vi "update gimbal.vi"(8 "error in \n(no error)":errorcluster, 10 "Current Position":T1, 11 "Data":T2) -> (0 "error out":errorcluster, 3 "Data":T2)   [LabVIEW 2015]
doc: "Artificial Horizon.VI\n\nRecieves Pitch Roll and Head, and using a 3D picture control Builds up an artifical horizon similar to that found in aircraft for example."
uses:
  typedefs/gimbal data.ctl
  <vilib>/Utility/miscctls.llb/LV3DPointTypeDef.ctl
  <vilib>/picture/3D Picture Control/NI_3D Picture Control.lvlib
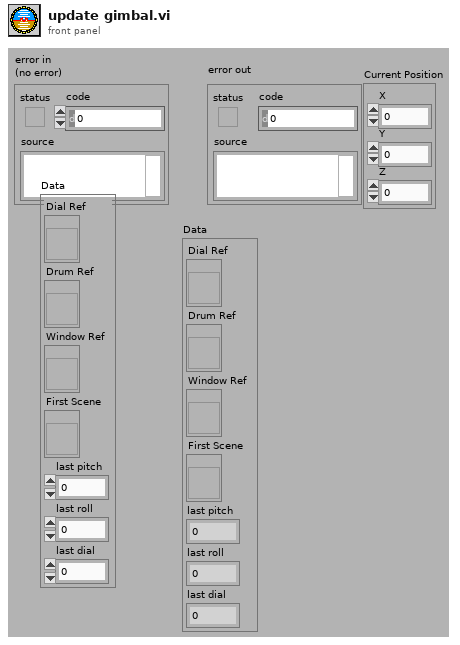
[diagram p1: front panel]
types:
  T1 = typedef "LV3DPointTypeDef.ctl" = cluster{"X":sgl, "Y":sgl, "Z":sgl}
  T2 = typedef "gimbal data.ctl" = cluster{"Dial Ref":refnum<vi>, "Drum Ref":refnum<vi>, "Window Ref":refnum<vi>, "First Scene":refnum<vi>, "last pitch":dbl, "last roll":dbl, "last dial":dbl}
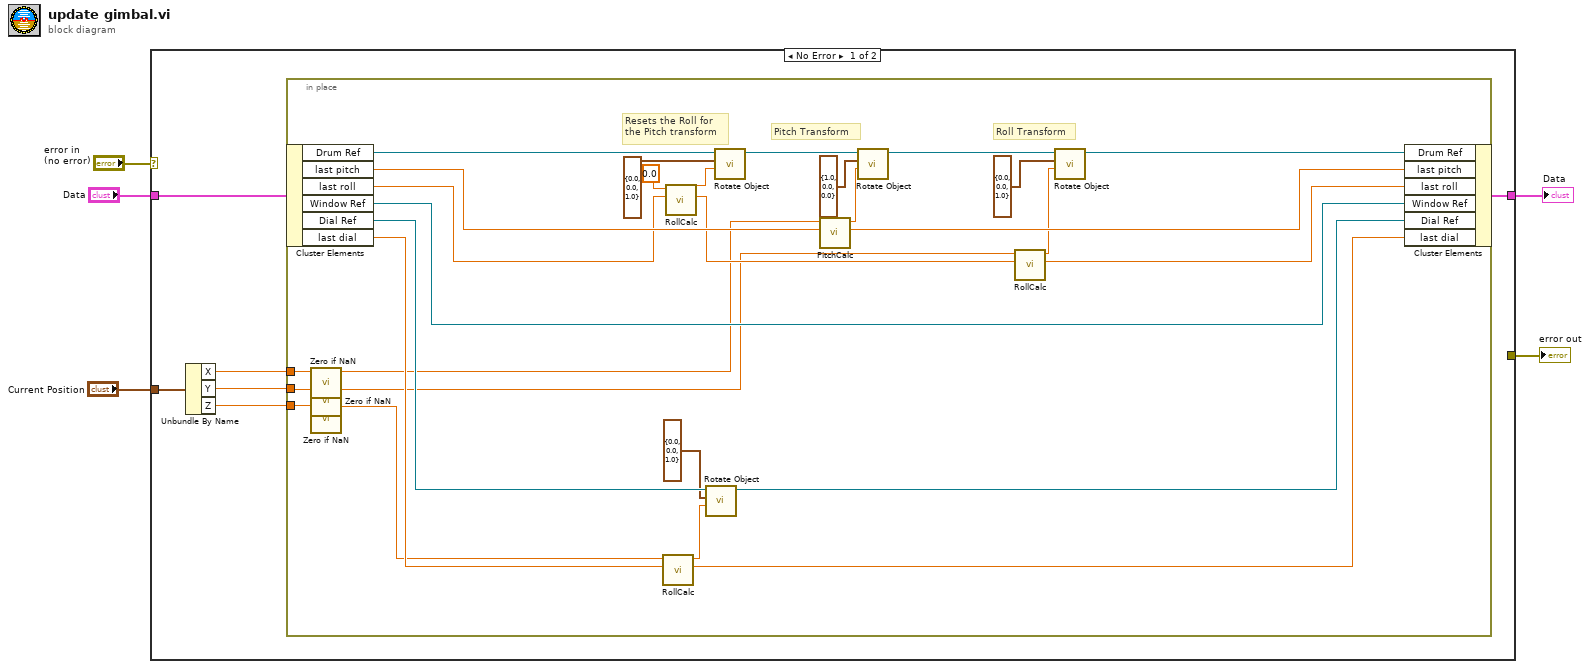
[diagram p0: block diagram]
diagram:
  n1 = case shown="No Error" "error in \n(no error)" {
    selector: "error in \n(no error)" -> [_ w42]
    tunnel: [_ w42] -> w4
    tunnel: "Data" -> [w11 w41]
    tunnel: [w10 w41] -> w2
    tunnel: "Current Position" -> [w9 _]
    frame No Error {
      n2 = Unbundle By Name(w9) -> ("X"=w8:sgl, "Y"=w7:sgl, "Z"=w6:sgl)
      n3 = in-place {
        in-place-border: w8 -> [w17]
        in-place-border: w7 -> [w15]
        in-place-border: w6 -> [w16]
        # "Roll Transform"
        # "Resets the Roll for \nthe Pitch transform"
        # "Pitch Transform"
        n4 = in-place-cluster #1(w11) -> ("Drum Ref"=w40:refnum<vi>, "last pitch"=w38:dbl, "last roll"=w36:dbl, "Window Ref"=w34:refnum<vi>, "Dial Ref"=w33:refnum<vi>, "last dial"=w31:dbl)
        n5 = call "Zero if NaN.vi"("Numeric"=w17) -> ("Numeric"=w14:dbl)  [unwired: 10 in]
        n6 = call "Zero if NaN.vi"("Numeric"=w15) -> ("Numeric"=w13:dbl)  [unwired: 10 in]
        n7 = call "Zero if NaN.vi"("Numeric"=w16) -> ("Numeric"=w12:dbl)  [unwired: 10 in]
        n8 = call "RollCalc.vi"("Previous Roll Value"=w31, "Roll Input"=w12) -> ("New Roll Value"=w30:dbl, "Adjustment to be Made"=w27:dbl)  [unwired: 8 in]
        n9 = call "RollCalc.vi"("Previous Roll Value"=w36, "Roll Input"=sgl 0.0 ("Angle")) -> ("New Roll Value"=w28:dbl, "Adjustment to be Made"=w22:dbl)  [unwired: 8 in]
        n10 = call <vilib>:"Rotate Object.vi"("Angle"=w27, "Axis"=cluster{"X":sgl, "Y":sgl, "Z":sgl} {"X"=0.0, "Y"=0.0, "Z"=1.0} ("Axis 2"), "Scene.Object In"=w33) -> ("Scene.Object Out"=w32:refnum<vi>)  [unwired: 7 in, 1 out]
        n11 = call <vilib>:"Rotate Object.vi"("Angle"=w22, "Axis"=cluster{"X":sgl, "Y":sgl, "Z":sgl} {"X"=0.0, "Y"=0.0, "Z"=1.0} ("Axis 2"), "Scene.Object In"=w40) -> ("Scene.Object Out"=w23:refnum<vi>)  [unwired: 7 in, 1 out]
        n12 = call "PitchCalc.vi"("Previous Pitch Value"=w38, "Pitch Control"=w14) -> ("New Pitch Value"=w37:dbl, "Adjustment to be made"=w24:dbl)  [unwired: 8 in]
        n13 = call <vilib>:"Rotate Object.vi"("Angle"=w24, "Axis"=cluster{"X":sgl, "Y":sgl, "Z":sgl} {"X"=1.0, "Y"=0.0, "Z"=0.0} ("Axis 2"), "Scene.Object In"=w23) -> ("Scene.Object Out"=w29:refnum<vi>)  [unwired: 7 in, 1 out]
        n14 = call "RollCalc.vi"("Previous Roll Value"=w28, "Roll Input"=w13) -> ("New Roll Value"=w35:dbl, "Adjustment to be Made"=w18:dbl)  [unwired: 8 in]
        n15 = call <vilib>:"Rotate Object.vi"("Angle"=w18, "Axis"=cluster{"X":sgl, "Y":sgl, "Z":sgl} {"X"=0.0, "Y"=0.0, "Z"=1.0} ("Axis 2"), "Scene.Object In"=w29) -> ("Scene.Object Out"=w39:refnum<vi>)  [unwired: 7 in, 1 out]
        n16 = in-place-cluster #1("Drum Ref"=w39, "last pitch"=w37, "last roll"=w35, "Window Ref"=w34, "Dial Ref"=w32, "last dial"=w30) -> (w10:T2)
      }
    }
    frame Error {
      # "OOOOOOOOOOOOOOOOOOOOOOOOOOO NNNNNNNNNNNNNNNNnnnnnnnnnnnnnnnnooooooooooooooooooooooooooooooooo\n\nAn Error..........................................................."
    }
  }
  "error out" <- w4
  "Data" <- w2
